vi "Load DAC Configuration.vi"(8 "error in":errorcluster, 10 "Config File refnum in":T1, 11 "DAC in":refnum<class "DAC.lvclass">) -> (0 "error out":errorcluster, 2 "Config File refnum out":T1, 3 "DAC out":refnum<class "DAC.lvclass">)   [LabVIEW 2019, in "DAC.lvlib" / "DAC.lvclass"]
uses:
  DAC.lvclass
  <vilib>/Utility/config.llb/Config Data RefNum.ctl
  DAC.lvclass/DAC.ctl
  <vilib>/Utility/config.llb/Read Key (Boolean).vi
  <vilib>/Utility/config.llb/Read Key (String).vi
  <vilib>/Utility/config.llb/Read Key (Double).vi
  <vilib>/Utility/config.llb/NI_LVConfig.lvlib
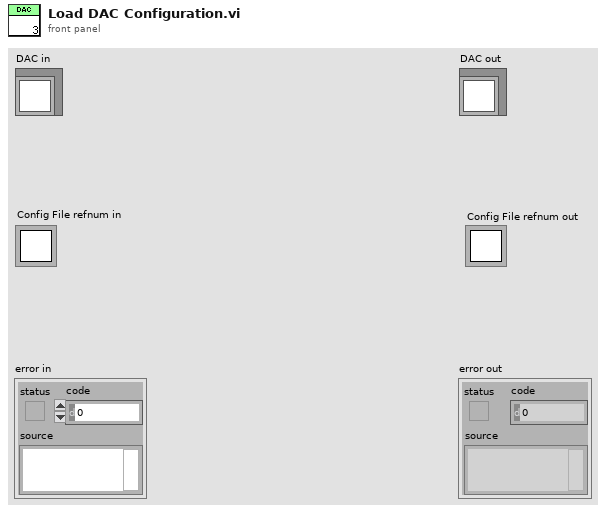
[diagram p1: front panel]
types:
  T1 = typedef "NI_LVConfig.lvlib/Config Data RefNum.ctl" = refnum<k1>
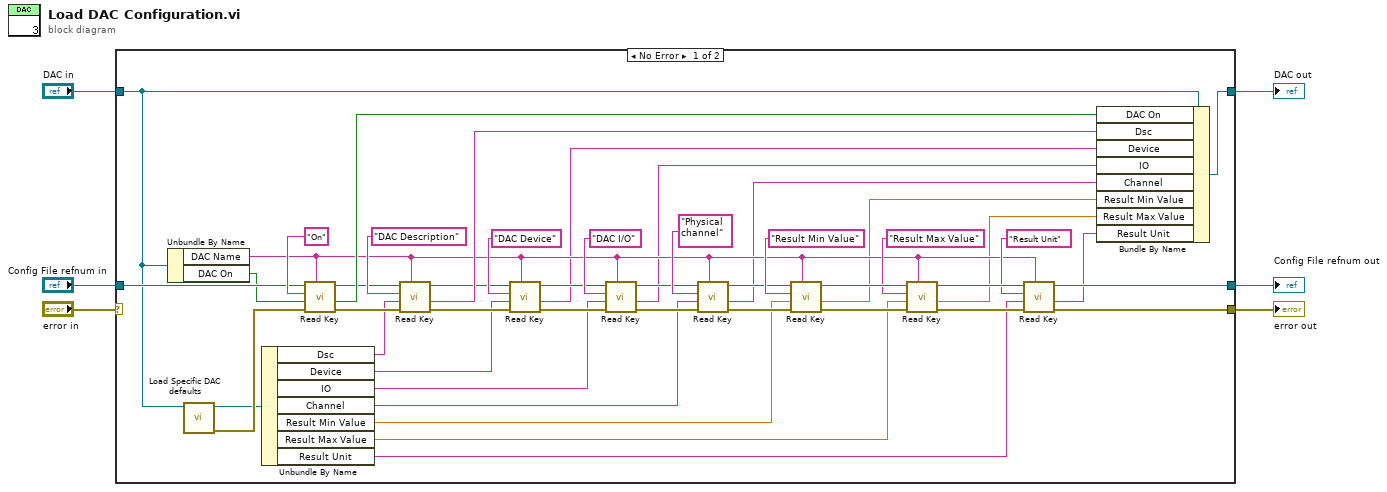
[diagram p0: block diagram]
diagram:
  n1 = case shown="No Error" "error in" {
    selector: "error in" -> [_ w55]
    tunnel: [w24 w55] -> w3
    tunnel: [w49 w54] -> w1
    tunnel: "DAC in" -> [w23 w54]
    tunnel: "Config File refnum in" -> [w51 w53]
    tunnel: [w25 w53] -> w2
    frame No Error {
      n2 = Unbundle By Name(w23) -> ("DAC Name"=w22:string, "DAC On"=w7:bool)
      n3 = call-dynamic "Load Specific DAC defaults.vi"("DAC in"=w23) -> ("error out"=w44:errorcluster, "DAC out"=w15:refnum<class "DAC.lvclass">)  [unwired: 9 in]
      n4 = Unbundle By Name(w15) -> ("Dsc"=w14:string, "Device"=w13:string, "IO"=w12:string, "Channel"=w11:string, "Result Min Value"=w10:dbl, "Result Max Value"=w9:dbl, "Result Unit"=w8:string)
      n5 = call-poly <vilib>:"Read Key.vi"("section"=w22, "error in (no error)"=w44, "default value"=w7, "key"="On", "refnum"=w51) -> ("error out"=w47:errorcluster, "value"=w50:bool, "refnum out"=w46:T1)  [unwired: 3 in, 1 out]
      n6 = call-poly <vilib>:"Read Key.vi"("section"=w22, "error in (no error)"=w47, "default value"=w14, "key"="DAC Description", "refnum"=w46) -> ("error out"=w28:errorcluster, "value"=w45:string, "refnum out"=w27:T1)  [unwired: 3 in, 1 out]
      n7 = call-poly <vilib>:"Read Key.vi"("section"=w22, "error in (no error)"=w28, "default value"=w13, "key"="DAC Device", "refnum"=w27) -> ("error out"=w29:errorcluster, "value"=w21:string, "refnum out"=w26:T1)  [unwired: 3 in, 1 out]
      n8 = call-poly <vilib>:"Read Key.vi"("section"=w22, "error in (no error)"=w29, "default value"=w12, "key"="DAC I/O", "refnum"=w26) -> ("error out"=w33:errorcluster, "value"=w20:string, "refnum out"=w34:T1)  [unwired: 3 in, 1 out]
      n9 = call-poly <vilib>:"Read Key.vi"("section"=w22, "error in (no error)"=w33, "default value"=w11, "key"="Physical channel", "refnum"=w34) -> ("error out"=w31:errorcluster, "value"=w19:string, "refnum out"=w32:T1)  [unwired: 3 in, 1 out]
      n10 = call-poly <vilib>:"Read Key.vi"("section"=w22, "error in (no error)"=w31, "default value"=w10, "key"="Result Min Value", "refnum"=w32) -> ("error out"=w41:errorcluster, "value"=w18:dbl, "refnum out"=w43:T1)  [unwired: 3 in, 1 out]
      n11 = call-poly <vilib>:"Read Key.vi"("section"=w22, "error in (no error)"=w41, "default value"=w9, "key"="Result Max Value", "refnum"=w43) -> ("error out"=w40:errorcluster, "value"=w17:dbl, "refnum out"=w42:T1)  [unwired: 3 in, 1 out]
      n12 = call-poly <vilib>:"Read Key.vi"("section"=w22, "error in (no error)"=w40, "default value"=w8, "key"="Result Unit", "refnum"=w42) -> ("error out"=w24:errorcluster, "value"=w16:string, "refnum out"=w25:T1)  [unwired: 3 in, 1 out]
      n13 = Bundle By Name(cluster=w23, "DAC On"=w50, "Dsc"=w45, "Device"=w21, "IO"=w20, "Channel"=w19, "Result Min Value"=w18, "Result Max Value"=w17, "Result Unit"=w16) -> (w49:refnum<class "DAC.lvclass">)
    }
    frame Error {
    }
  }
  "error out" <- w3
  "DAC out" <- w1
  "Config File refnum out" <- w2
